vi "Write Stored Sessions.vi"(10 "Stored Sessions":refnum<class "Session.lvclass">[](array[class]), 11 "ConnectionHandler in":refnum<class "ConnectionHandler.lvclass">) -> (3 "ConnectionHandler":refnum<class "ConnectionHandler.lvclass">)   [LabVIEW 2013, in "MQTT_Connection.lvlib" / "ConnectionHandler.lvclass"]
uses:
  ConnectionHandler.lvclass
  MQTT_Base/Session/Session.lvclass
  ConnectionHandler.lvclass/ConnectionHandler.ctl
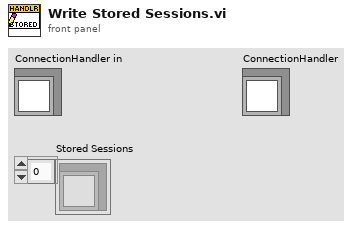
[diagram p1: front panel]
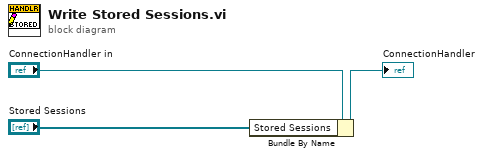
[diagram p0: block diagram]
diagram:
  n1 = Bundle By Name(cluster="ConnectionHandler in", "Stored Sessions"="Stored Sessions") -> (→"ConnectionHandler":refnum<class "ConnectionHandler.lvclass">)
